vi "BasicReadoutV830.vi"() -> ()   [LabVIEW 2014]
uses:
  Program Files (x86)/CAEN/Comm/labview/CAENComm.lvlib
panel:
  out "Raw Data":u32[](array[numeric])
  in  "stop":bool
  in  "VME Base Address":u32=4026662912 format="%.0x"
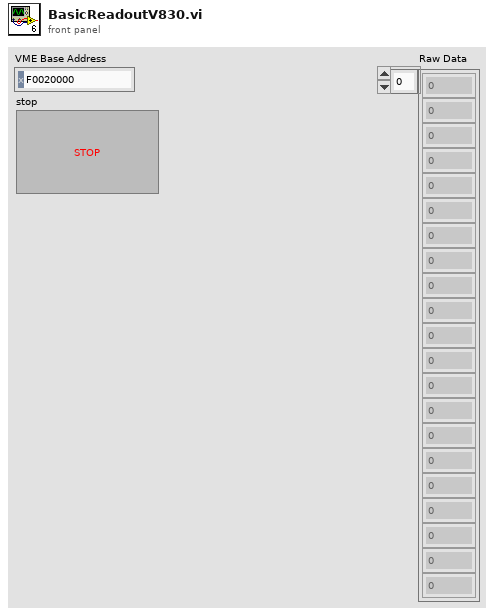
[diagram p1: front panel]
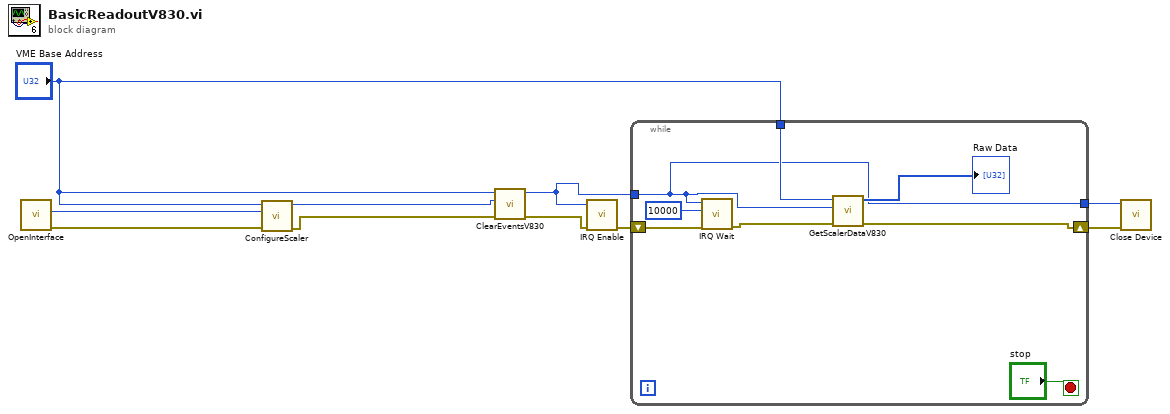
[diagram p0: block diagram]
diagram:
  n1 = call "OpenInterface.vi"() -> ("error out"=w4:errorcluster, "handle"=w6:i32)  [unwired: 9 in, 1 out]
  n2 = call "ConfigureScaler.vi"("error in (no error)"=w4, "handle"=w6, "VME Base Address"="VME Base Address") -> ("error out"=w3:errorcluster, "handle out"=w2:i32)  [unwired: 6 in, 1 out]
  n3 = call "ClearEventsV830.vi"("error in (no error)"=w3, "handle in"=w2, "VME Base Address"="VME Base Address") -> ("error out"=w10:errorcluster, "handle out"=w1:i32)  [unwired: 7 in]
  n4 = call "IRQ Enable.vi"("error in (no error)"=w10, "handle"=w1) -> ("error out"=w9:errorcluster)  [unwired: 9 in]
  n5 = while {
    shift-right: [w14] -> w8
    shift-left: w9 -> [w16]
    tunnel: w1 -> [w11]
    tunnel: [w11] -> w7
    tunnel: "VME Base Address" -> [w12]
    stop <- "stop" stop-if-true
    n6 = call "IRQ Wait.vi"("error in (no error)"=w16, "Timeout"=u32 10000, "handle"=w11) -> ("error out"=w13:errorcluster)  [unwired: 8 in]
    n7 = call "GetScalerDataV830.vi"("error in (no error)"=w13, "handle in"=w11, "VME Base Address"=w12) -> ("error out"=w14:errorcluster, "Buff"=→"Raw Data":u32[])  [unwired: 6 in, 1 out]
  }
  n8 = call "Close Device.vi"("error in (no error)"=w8, "handle"=w7) -> ()  [unwired: 9 in, 1 out]
